vi "Robot Global Data.vi"() -> ()   [LabVIEW 2023]
doc: "This global VI can contain as many global variables as you need. To create a global variable, place a control on the panel, give it a good name. To read or write to it from a VI, drag the icon to the diagram of that VI. You can also drag from the project. Click on the node to change which global you access. You shouldn't have multiple locations writing to a global or it will cause a race-condition."
uses:
  <vilib>/Rock Robotics/WPI/Camera/WPI_CameraImageSize.ctl
  <vilib>/Rock Robotics/WPI/DriverStation/WPI_DriverStationRobotMode2.ctl
  Drive/Implementation/Drive Setpoints.ctl
  Drive/Implementation/Drive Operations.ctl
  swerve/Type Definitions/Data/Robot Velocities.ctl
  <vilib>/Rock Robotics/WPI/Framework/Command Status Info.ctl
  <vilib>/Rock Robotics/WPI/Framework/Completion Status.ctl
  <vilib>/Rock Robotics/WPI/Framework/Completion Notifier.ctl
  swerve/Type Definitions/Data/Pod Positions.ctl
  <vilib>/Rock Robotics/WPI/MotorControl/WPI_MotorControlDeviceRef.ctl
  <vilib>/Rock Robotics/WPI/MotorControl/WPI_MotorControlType.ctl
  <vilib>/Rock Robotics/SystemInterfaces/DIO/FPGA_DIOPWMChannel.ctl
  <vilib>/Rock Robotics/WPI/PWM/WPI_PWMDeadband.ctl
  <vilib>/Rock Robotics/SystemInterfaces/DIO/FPGA_DIOChannel.ctl
panel:
  in  "Vision Start":dbl
  in  "Cascade Raise Times":T1={"Trough"=1.0, "L2"=1.0, "L3"=1.7, "L4"=2.2}
  in  "Align Button Pressed?":bool
  in  "Sees Reef?":bool=TRUE
  in  "Climb Coast":bool
  in  "Has Coral?":bool
  in  "Can Cascade?":bool
  in  "Robot Velocities":T2={"X Velocity"=0.0, "Y Velocity"=-0.0, "Rotational \nVelocity"=-0.0}
  in  "Aligning?":bool
  in  "Can Climb?":bool
  in  "Have Ball?":bool
  in  "Motor Data":T3[](array[typedef])
  in  "Pod Radius":dbl=0.9375
  out "Pod Locations":T8 {"Right Back Position" format="%.2f"; "Right Front Position" format="%.2f"; "Left Back Position" format="%.2f"; "Left Front Position" format="%.2f"}
  out "Drive Controller Data":T14={"SubSystem Data"={"Operation"=enum."Immediate", "Robot Velocities"={"X Velocity"=0.0, "Y Velocity"=-0.0, "Rotational \nVelocity"=-0.0}, "Auto Data"={"Auto Velocities"=[], "Auto Positions"=[], "Auto Commands"=[], "Zero Velocity?"=[]}, "Left side"=FALSE, "Angle Align"=FALSE, "Tag ID"=0}, {"Start Time (ms)"=7747115, "Iterations"=0}, {"Command Info"={"Name"="", "Status"=enum."Successful", "notifier out"=refnum}, "Description"="", "Default Command"={"Operation"=enum."Reserve", "Robot Velocities"={"X Velocity"=0.0, "Y Velocity"=0.0, "Rotational \nVelocity"=0.0}, "Auto Data"={"Auto Velocities"=[], "Auto Positions"=[], "Auto Commands"=[], "Zero Velocity?"=[]}, "Left side"=FALSE, "Angle Align"=FALSE, "Tag ID"=0}, "queue out"=refnum, "Subsystem Name"="Drive"}}
  in  "Auto Done?":bool
  in  "Drive Conditions":T15={"Field Centric"=TRUE, "Reef Centric"=FALSE}
  in  "Robot Mode":T16=enum."Teleop Enabled"
  in  "image size":T17=enum."320x240"
  in  "Enable Vision":bool
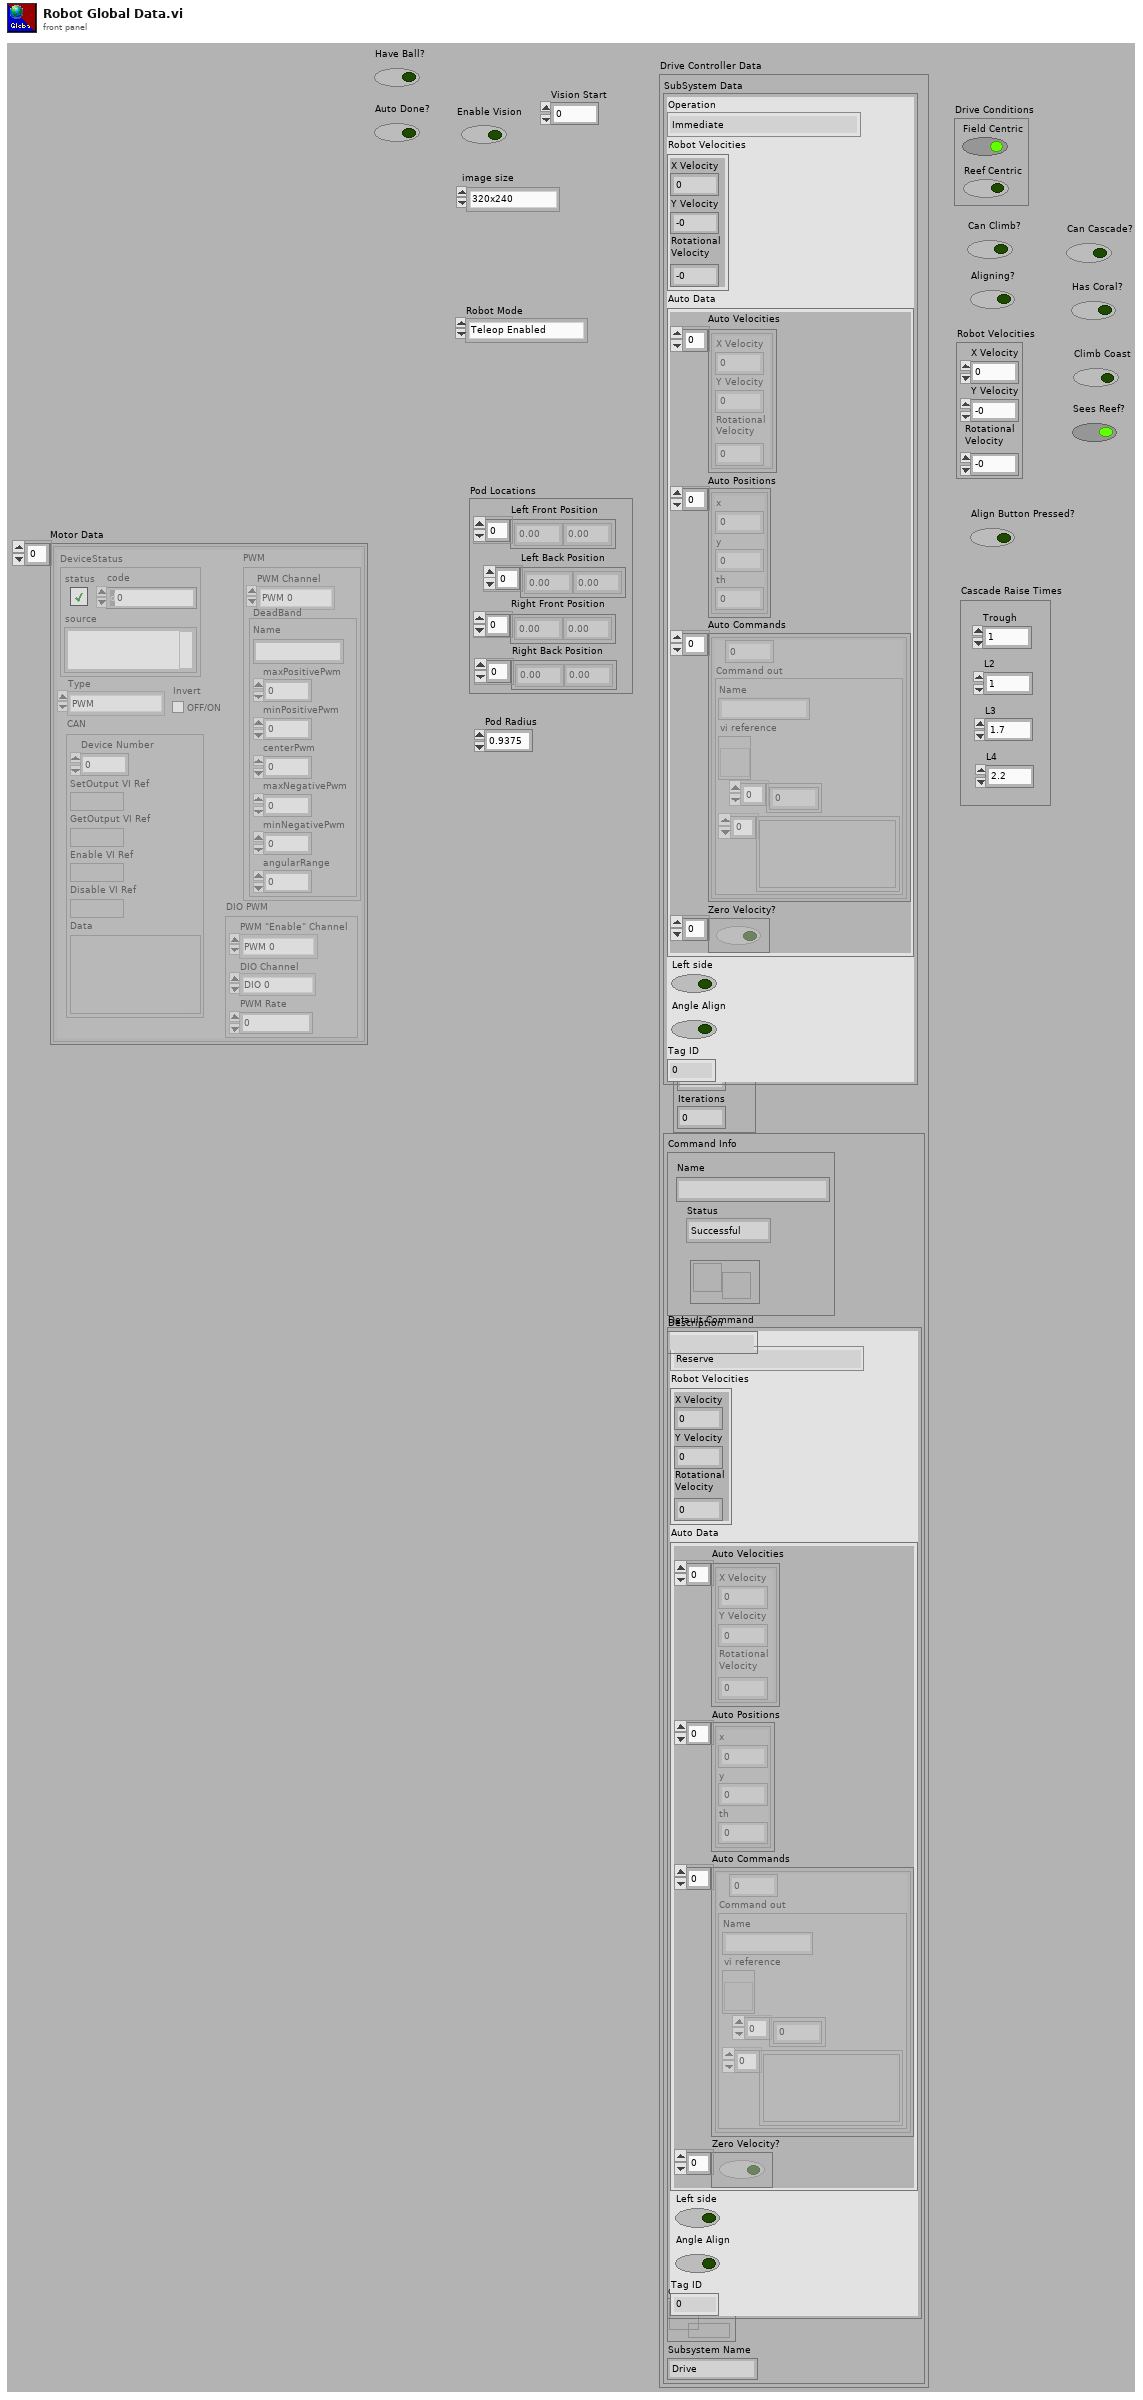
[diagram p1: front panel]
types:
  T1 = cluster{"Trough":dbl, "L2":dbl, "L3":dbl, "L4":dbl}
  T2 = typedef "Robot Velocities.ctl" = cluster{"X Velocity":dbl, "Y Velocity":dbl, "Rotational \nVelocity":dbl}
  T3 = typedef "WPI_MotorControlDeviceRef.ctl" = cluster{"DeviceStatus":errorcluster, "Type":T4, "PWM":cluster{"PWM Channel":T5, "DeadBand":T6}, "CAN":cluster{"Device Number":u8, "SetOutput VI Ref":variant, "GetOutput VI Ref":variant, "Enable VI Ref":variant, "Disable VI Ref":variant, "Data":variant}, "Invert":bool, "DIO PWM":cluster{"PWM \"Enable\" Channel":T5, "DIOChannel":T7, "PWM Rate":dbl}}
  T4 = typedef "WPI_MotorControlType.ctl" = enum16{"PWM", "CAN", "DIO PWM"}
  T5 = typedef "FPGA_DIOPWMChannel.ctl" = enum8{"PWM 0", "PWM 1", "PWM 2", "PWM 3", "PWM 4", "PWM 5", "PWM 6", "PWM 7", "PWM 8", "PWM 9", "PWM MXP 0", "PWM MXP 1", "PWM MXP 2", "PWM MXP 3", "PWM MXP 4", "PWM MXP 5", "PWM MXP 6", "PWM MXP 7", "PWM MXP 8", "PWM MXP 9", "Invalid"}
  T6 = typedef "WPI_PWMDeadband.ctl" = cluster{"Name":string, "maxPositivePwm":i32, "minPositivePwm":i32, "centerPwm":i32, "maxNegativePwm":i32, "minNegativePwm":i32, "angularRange":u16}
  T7 = typedef "FPGA_DIOChannel.ctl" = enum8{"DIO 0", "DIO 1", "DIO 2", "DIO 3", "DIO 4", "DIO 5", "DIO 6", "DIO 7", "DIO 8", "DIO 9", "DIO MXP 0", "DIO MXP 1", "DIO MXP 2", "DIO MXP 3", "DIO MXP 4", "DIO MXP 5", "DIO MXP 6", "DIO MXP 7", "DIO MXP 8", "DIO MXP 9", "DIO MXP 10", "DIO MXP 11", "DIO MXP 12", "DIO MXP 13", "DIO MXP 14", "DIO MXP 15", "SPI Port CS1", "SPI Port CS2", "SPI Port CS3", "SPI Port MISO", "SPI Port MOSI", "Invalid"}
  T8 = typedef "Pod Positions.ctl" = cluster{"Left Front Position":dbl[], "Left Back Position":dbl[], "Right Front Position":dbl[], "Right Back Position":dbl[]}
  T9 = typedef "Drive Setpoints.ctl" = cluster{"Operation":T10, "Robot Velocities":T2, "Auto Data":cluster{"Auto Velocities":T2[], "Auto Positions":cluster{"x":dbl, "y":dbl, "th":dbl}[], "Auto Commands":cluster{dbl, "Command out":cluster{"Name":string, "vi reference":refnum<vi>, i32[], variant[]}}[], "Zero Velocity?":bool[]}, "Left side":bool, "Angle Align":bool, "Tag ID":i32}
  T10 = typedef "Drive Operations.ctl" = enum16{"Reserve", "Read Current", "Immediate", "Calibrate", "Reef Align", "Auto"}
  T11 = typedef "Command Status Info.ctl" = cluster{"Name":string, "Status":T12, "notifier out":T13}
  T12 = typedef "Completion Status.ctl" = enum16{"Successful", "Aborted", "Incomplete"}
  T13 = typedef "Completion Notifier.ctl" = refnum<notifier>
  T14 = cluster{"SubSystem Data":T9, cluster{"Start Time (ms)":u32, "Iterations":i32}, cluster{"Command Info":T11, "Description":string, "Default Command":T9, "queue out":refnum<queue>, "Subsystem Name":string}}
  T15 = cluster{"Field Centric":bool, "Reef Centric":bool}
  T16 = typedef "WPI_DriverStationRobotMode2.ctl" = enum16{"Autonomous Disabled", "Autonomous Enabled", "Teleop Disabled", "Teleop Enabled", "Disconnected", "Finish", "Test Disabled", "Test Enabled", "Emergency Stopped"}
  T17 = typedef "WPI_CameraImageSize.ctl" = enum16{"640x480", "320x240", "160x120", "Custom"}
diagram:
